vi "DisplayData.vi"(8 "前面板窗口:标题":string, 9 "变体":variant) -> ()   [LabVIEW 2020]
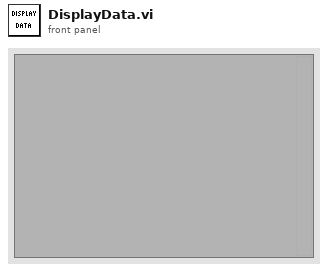
[diagram p1: front panel]
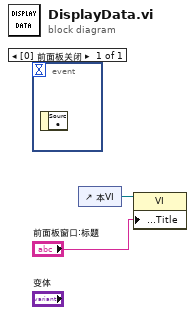
[diagram p0: block diagram]
diagram:
  n1 = event shown="[0] 前面板关闭" {
    selector: _ -> [_]
    dyn-events: _ -> [_]
    timeout: _ -> [_]
    event Panel Close {
      n2 = event-data() -> ()  [unwired: 1 in, 1 out]
    }
  }
  n3 = control-ref of="本VI"() -> (w2:refnum<vi>)
  n4 = property class="VI"(reference=w2, "Front Panel.Title"="前面板窗口:标题") -> ()  [unwired: 1 in, 2 out]
